vi "Main.vi"() -> ()   [LabVIEW 2019]
uses:
  <vilib>/Analysis/2dsp.llb/Real FFT.vi
  <vilib>/Analysis/NI_AALPro.lvlib
panel:
  out "Cursor values":dbl[][](array[numeric])
  in  "Export Button":bool
  in  "Count":i32=3
  in  "Stop Button":bool
  out "Waveform Graph":dbl[](graph)
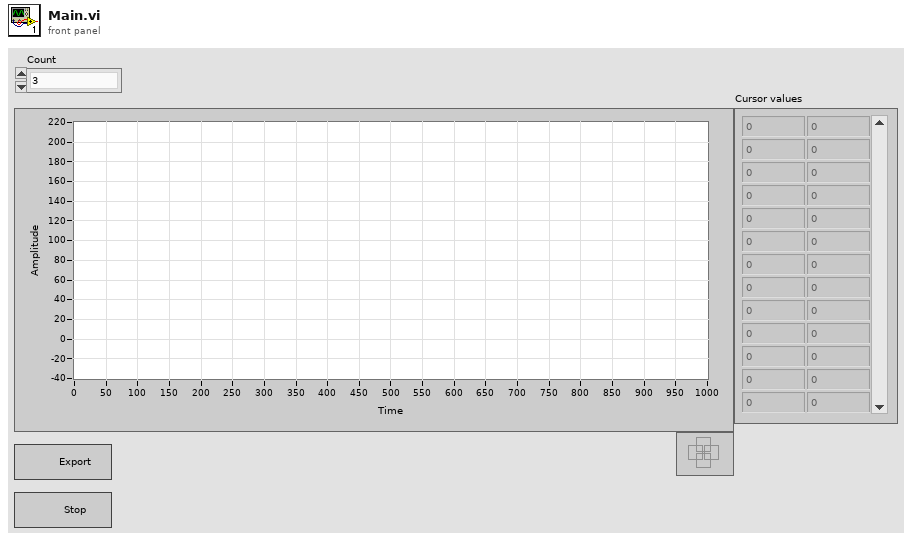
[diagram p1: front panel]
types:
  T1 = cluster{"Name":string, "Color":u32, "Style":i32, "Point Style":u8, "Name Visible":bool, "Allow Drag":bool, "Cursor Mode":u32, "Plot":i32, "Index":i32, "Position":cluster{"X":dbl, "Y":dbl}, "X Scale":u32, "Y Scale":u32, "Watch Plots":i32[], "Watch All Plots":bool, "Plot Area":i32, "Label Offset":cluster{"X":dbl, "Y":dbl}}
  T2 = cluster{"Name":string, "Color":u32, "Style":i32, "Point Style":u8, "Name Visible":bool, "Allow Drag":bool, "Cursor Mode":u32, "Plot":i32, "Index":i32, "Position":cluster{"X":dbl, "Y":dbl}, "X Scale":u32, "Y Scale":u32, "Watch Plots":i32[], "Watch All Plots":bool, "Plot Area":i32, "Label Offset":cluster{"X":dbl, "Y":dbl}}[]
  T3 = typedef "LVCursorListTypeDef.ctl" = cluster{"Name":string, "Color":u32, "Style":u8, "Point Style":u8, "Name Visible":bool, "Allow Drag":bool, "Cursor Mode":u32, "Plot":i32, "Index":i32, "Position":cluster{"X":dbl, "Y":dbl}, "X Scale":u32, "Y Scale":u32, "Watch Plots":i32[], "Watch All Plots":bool, "Plot Area":i32, "Label Offset":cluster{"X":dbl, "Y":dbl}}[]
  T4 = cluster{"Name":string, "Color":u32, "Style":u8, "Point Style":u8, "Name Visible":bool, "Allow Drag":bool, "Cursor Mode":u32, "Plot":i32, "Index":i32, "Position":cluster{"X":dbl, "Y":dbl}, "X Scale":u32, "Y Scale":u32, "Watch Plots":i32[], "Watch All Plots":bool, "Plot Area":i32, "Label Offset":cluster{"X":dbl, "Y":dbl}}
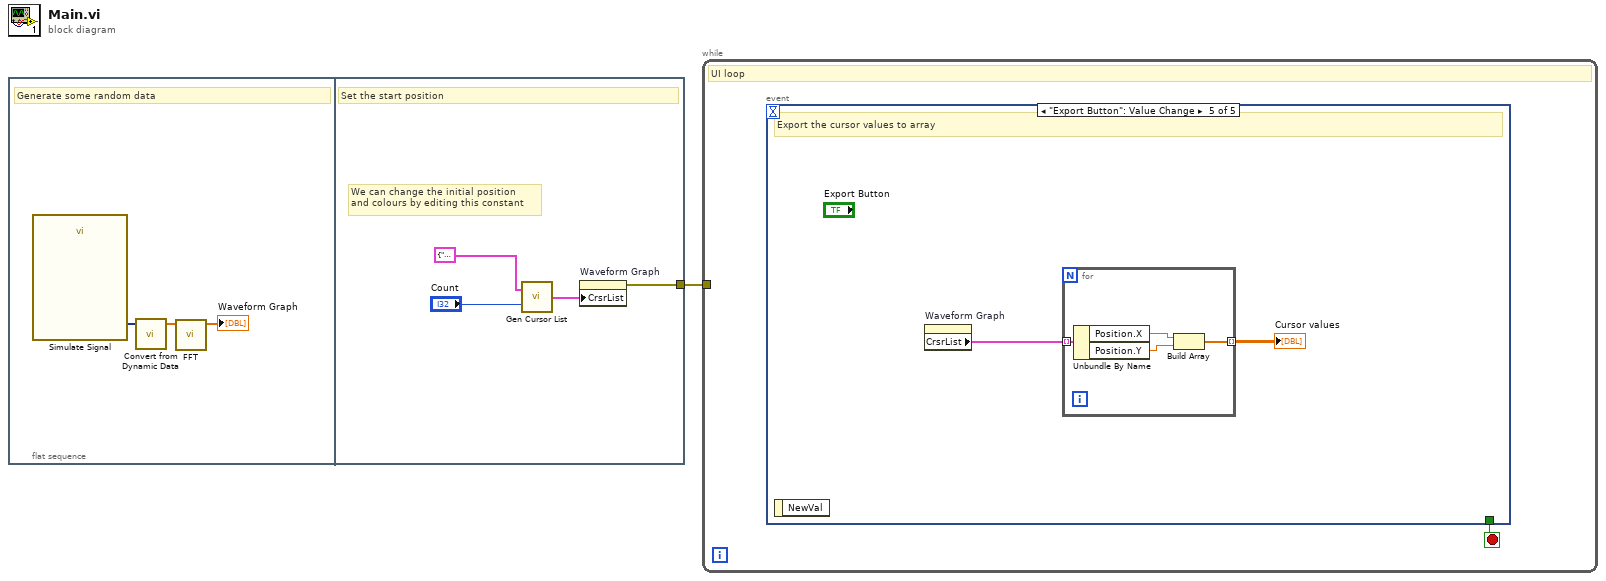
[diagram p0: block diagram]
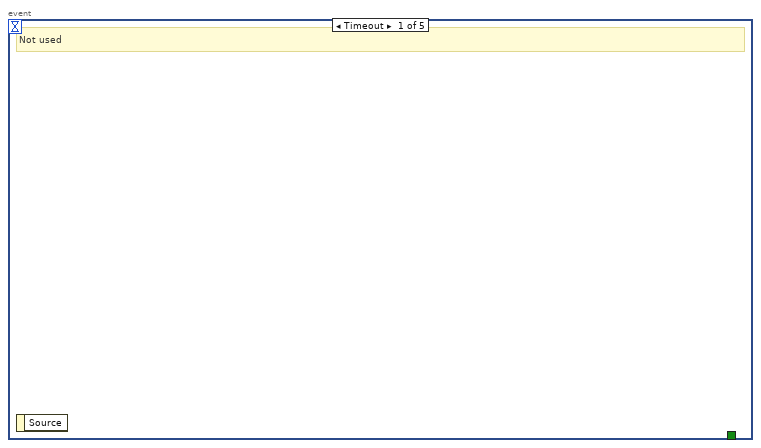
[diagram p2: hidden frame]
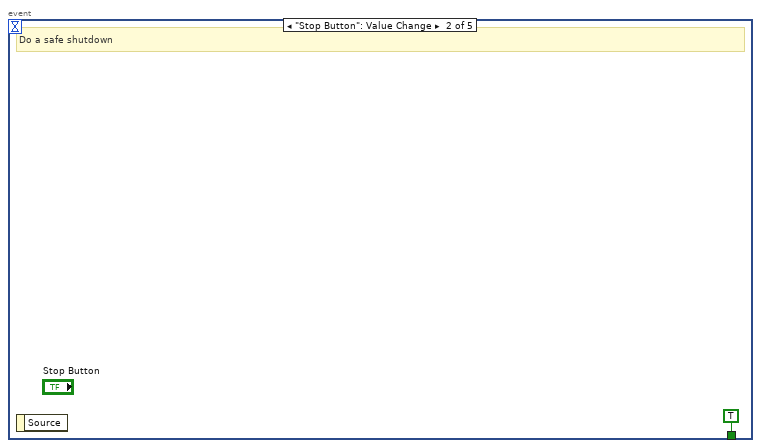
[diagram p3: hidden frame]
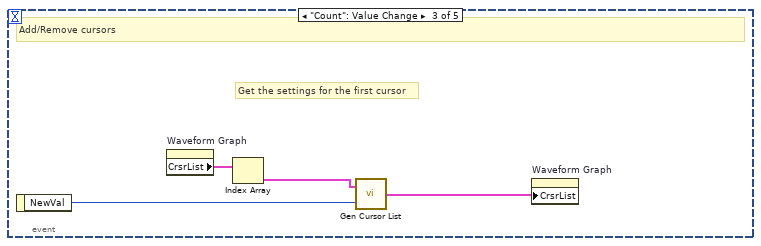
[diagram p4: hidden frame]
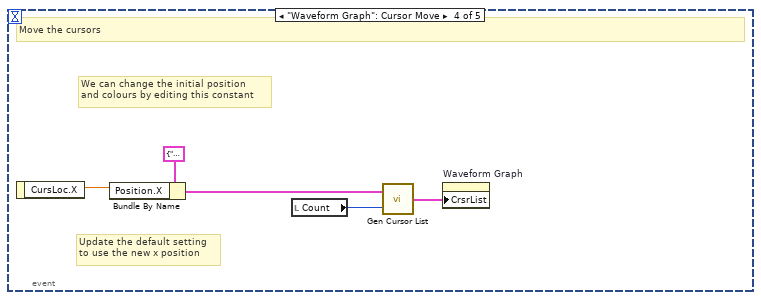
[diagram p5: hidden frame]
diagram:
  n1 = flat-sequence {
    tunnel: [w7] -> w1
    frame #0 {
      # "Generate some random data"
      n2 = call "Simulate Signal"() -> ("Square with Uniform Noise"=w4:dynamicdata)  [unwired: 14 in, 1 out]
      n3 = call "Convert from Dynamic Data"("Dynamic Data Type"=w4) -> ("Array"=w3:dbl[])  [unwired: 3 in]
      n4 = call-poly <vilib>:"FFT.vi"("X"=w3) -> ("FFT {X}"=→"Waveform Graph":cdb[])  [unwired: 9 in, 1 out]
    }
    frame #1 {
      # "We can change the initial position \nand colours by editing this constant"
      # "Set the start position"
      n5 = call "Gen Cursor List.vi"("Count in"="Count", "Settings in"=T1 {"Name"="Cursor 0", "Color"=16711680, "Style"=2, "Point Style"=13, "Name Visible"=FALSE, "Allow Drag"=TRUE, "Cursor Mode"=1, "Plot"=-1, "Index"=310, "Position"={"X"=50.1, "Y"=0.0}, "X Scale"=0, "Y Scale"=0, "Watch Plots"=[], "Watch All Plots"=FALSE, "Plot Area"=0, "Label Offset"={"X"=-0.00649752475247567, "Y"=6.211909771510491}}) -> ("CrsrLst Out"=w8:T2)
      n6 = property on="Waveform Graph" class="WFGraph (strict)"("CrsrList"=w8) -> (error out=w7:errorcluster)  [unwired: 2 in, 1 out]
    }
  }
  n7 = while {
    tunnel: w1 -> [_]
    stop <- w9 stop-if-true
    # "UI loop"
    n8 = event shown="[4] \"Export Button\": Value Change" {
      selector: _ -> [_ _ _ _ _]
      dyn-events: _ -> [_ _ _ _ _]
      timeout: _ -> [_ _ _ _ _]
      tunnel: [_ TRUE _ _ _] -> w9
      event Timeout {
        # "Not used"
        n9 = event-data() -> ()  [unwired: 1 in, 1 out]
      }
      event "Stop Button": Value Change {
        # "Do a safe shutdown"
        n10 = event-data() -> ()  [unwired: 1 in, 1 out]
      }
      event "Count": Value Change {
        # "Get the settings for the first cursor"
        # "Add/Remove cursors"
        n11 = event-data() -> ("NewVal"=w12:i32)  [unwired: 1 in]
        n12 = property on="Waveform Graph" class="WFGraph (strict)"() -> ("CrsrList"=w14:T3)  [unwired: 2 in, 2 out]
        n13 = Index Array(array=w14) -> (element=w13:T4)  [unwired: 1 in]
        n14 = call "Gen Cursor List.vi"("Count in"=w12, "Settings in"=w13) -> ("CrsrLst Out"=w11:T2)
        n15 = property on="Waveform Graph" class="WFGraph (strict)"("CrsrList"=w11) -> ()  [unwired: 2 in, 2 out]
      }
      event "Waveform Graph": Cursor Move {
        # "Update the default setting \nto use the new x position"
        # "We can change the initial position \nand colours by editing this constant"
        # "Move the cursors"
        n16 = event-data() -> ("CursLoc.X"=w18:dbl)  [unwired: 1 in]
        n17 = Bundle By Name(cluster=T1 {"Name"="Cursor 0", "Color"=16711680, "Style"=2, "Point Style"=13, "Name Visible"=FALSE, "Allow Drag"=TRUE, "Cursor Mode"=1, "Plot"=-1, "Index"=310, "Position"={"X"=50.1, "Y"=0.0}, "X Scale"=0, "Y Scale"=0, "Watch Plots"=[], "Watch All Plots"=FALSE, "Plot Area"=0, "Label Offset"={"X"=-0.00649752475247567, "Y"=6.211909771510491}}, "Position.X"=w18) -> (w17:T1)
        n18 = local read "Count"() -> (w16:i32)
        n19 = call "Gen Cursor List.vi"("Count in"=w16, "Settings in"=w17) -> ("CrsrLst Out"=w15:T2)
        n20 = property on="Waveform Graph" class="WFGraph (strict)"("CrsrList"=w15) -> ()  [unwired: 2 in, 2 out]
      }
      event "Export Button": Value Change {
        # "Export the cursor values to array"
        n21 = event-data() -> ()  [unwired: 1 in, 1 out]
        n22 = property on="Waveform Graph" class="WFGraph (strict)"() -> ("CrsrList"=w21:T3)  [unwired: 2 in, 2 out]
        n23 = for {
          tunnel: w21 -> [w25] mode=indexing
          tunnel: [w22] -> w20 mode=indexing
          n24 = Unbundle By Name(w25) -> ("Position.X"=w24:dbl, "Position.Y"=w23:dbl)
          n25 = Build Array(w24, w23) -> (w22:dbl[])
        }
        "Cursor values" <- w20
      }
    }
  }
